vi "Get node version Q.vi"(11 "error in":errorcluster) -> (8 "LEIN custom reply Q":T1, 15 "error out":errorcluster)   [LabVIEW 2011]
uses:
  Defenitions/LEIN custom reply Q.ctl
  Defenitions/LEIN Reply Holder.ctl
  Defenitions/LEIN CMD Cluster.ctl
  Defenitions/LEIN CMD List.ctl
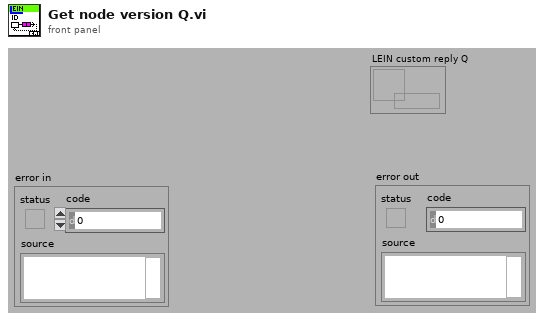
[diagram p1: front panel]
types:
  T1 = typedef "LEIN custom reply Q.ctl" = refnum<queue>
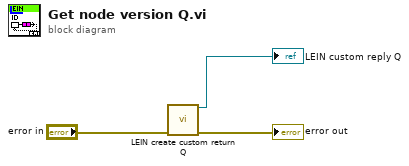
[diagram p0: block diagram]
diagram:
  n1 = call "LEIN create custom return Q.vi"("error in (no error)"="error in") -> ("LEIN custom reply Q"=→"LEIN custom reply Q":T1, "error out"=→"error out":errorcluster)  [unwired: 13 in]
